vi "DBConnect.vi"(8 "error in (no error)":errorcluster, 11 "connection path":path) -> (0 "error out":errorcluster, 3 "db connection out":T1)   [LabVIEW 2016]
uses:
  <vilib>/addons/database/Connection.llb/Conn ObjectReference.ctl
  <vilib>/addons/database/Connection.llb/DB Tools Open Connec (Path).vi
  <vilib>/addons/database/NI_Database_API.lvlib
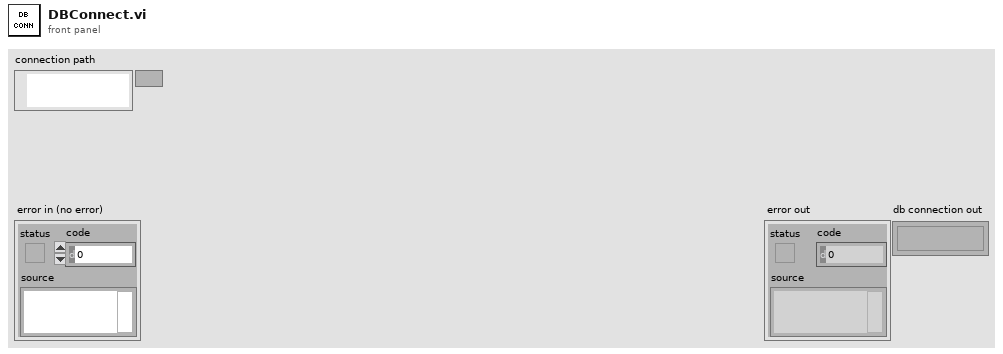
[diagram p1: front panel]
types:
  T1 = typedef "NI_Database_API.lvlib/Conn ObjectReference.ctl" = refnum<k1>
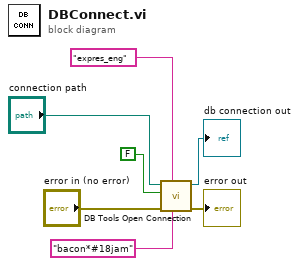
[diagram p0: block diagram]
diagram:
  n1 = call-poly <vilib>:"DB Tools Open Connection.vi"("password"="bacon*#18jam", "userID"="expres_eng", "error in (no error)"="error in (no error)", "prompt? (F)"=FALSE, "connection information"="connection path") -> ("error out"=→"error out":errorcluster, "connection reference"=→"db connection out":T1)  [unwired: 3 in]
